vi "Script PD.vi"(6 "PD Cluster":refnum<vi>, 8 "error in":errorcluster, 9 "PD Control":refnum<vi>, 10 "Terminal Attributes":T1) -> (0 "error out":errorcluster)   [LabVIEW 2025, in "_Rescript.lvlib" / "_Rescript.lvclass"]
uses:
  _Rescript.lvclass
  _Rescript.lvclass/_Rescript.ctl
  _Rescript.lvlib
  Attributes.ctl
  Terminal Attributes.ctl
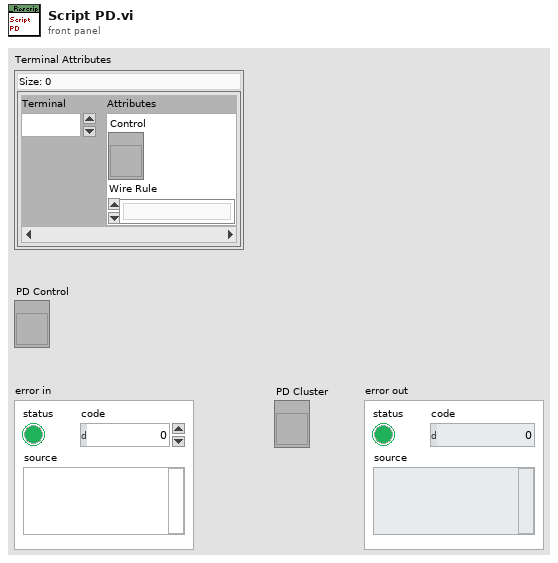
[diagram p1: front panel]
types:
  T1 = typedef "_Rescript.lvlib/Terminal Attributes.ctl" = map{i32, T2}
  T2 = typedef "_Rescript.lvlib/Attributes.ctl" = cluster{"Control":refnum<vi>, "Wire Rule":enum16{"Invalid Wire Rule", "Required", "Recommended", "Optional", "Dynamic Dispatch"}}
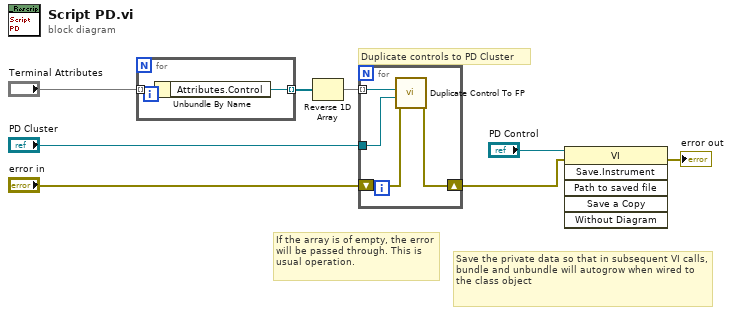
[diagram p0: block diagram]
diagram:
  # "If the array is of empty, the error will be passed through. This is usual operation."
  # "Duplicate controls to PD Cluster"
  # "Save the private data so that in subsequent VI calls, bundle and unbundle will autogrow when wired to the class object"
  n1 = for {
    tunnel: "Terminal Attributes" -> [w10] mode=indexing
    tunnel: [w9] -> w2 mode=indexing
    n2 = Unbundle By Name(w10) -> ("Attributes.Control"=w9:refnum<vi>)
  }
  n3 = Reverse 1D Array(array=w2) -> (reversed array=w1:refnum<vi>[])
  n4 = for {
    tunnel: "PD Cluster" -> [w13]
    shift-right: [w11] -> w4
    shift-left: "error in" -> [w12]
    tunnel: w1 -> [w14] mode=indexing
    n5 = call "Duplicate Control To FP.vi"("error in"=w12, "Owner"=w13, "Control"=w14) -> ("error out"=w11:errorcluster)  [unwired: 8 in]
  }
  n6 = invoke class="VI" method="Save.Instrument"(reference="PD Control", error in=w4) -> (error out=→"error out":errorcluster)  [unwired: 4 in, 5 out]
